vi "Get Meter Selected.vi"(0 "VISA resource name":refnum<visa-resource-name>, 11 "error in (no error)":errorcluster) -> (4 "VISA resource name out":refnum<visa-resource-name>, 6 "Meter Selected":u16(ring) items=["Frequency", "Peak Current", "Power", "Current", "Power Factor"], 15 "error out":errorcluster)   [LabVIEW 2020, in "eec 6700.lvlib"]
doc: "Gets the current meter selected in the power source instrument."
uses:
  <instrlib>/eec 6700/eec 6700.lvlib
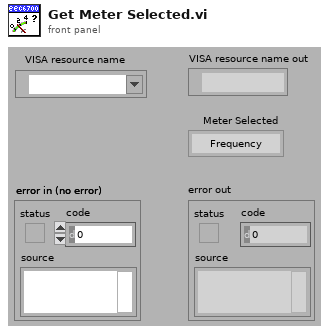
[diagram p1: front panel]
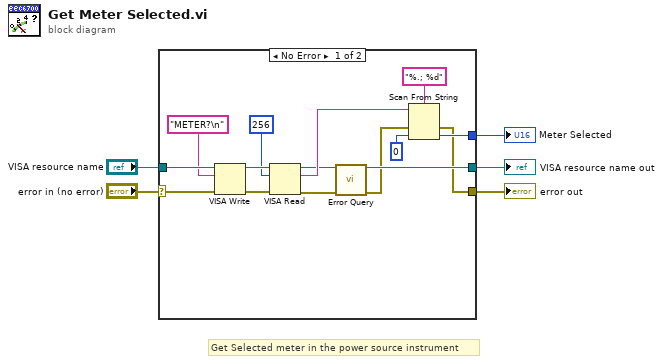
[diagram p0: block diagram]
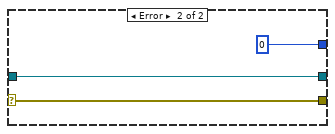
[diagram p2: hidden frame]
diagram:
  # "Get Selected meter in the power source instrument"
  n1 = case shown="No Error" "error in (no error)" {
    selector: "error in (no error)" -> [w11 w23]
    tunnel: "VISA resource name" -> [w20 w22]
    tunnel: [w10 w22] -> w4
    tunnel: [w8 w23] -> w3
    tunnel: [w15 u16 0 ("default value 1")] -> w2
    frame No Error {
      n2 = VISA Write(VISA resource name=w20, write buffer="METER?\n" ("command"), error in (no error)=w11) -> (VISA resource name out=w19:refnum<visa-resource-name>, error out=w18:errorcluster)  [unwired: 1 out]
      n3 = VISA Read(VISA resource name=w19, byte count=u32 256, error in (no error)=w18) -> (VISA resource name out=w9:refnum<visa-resource-name>, read buffer=w12:string, error out=w6:errorcluster)  [unwired: 1 out]
      n4 = call <instrlib>:"Error Query.vi"("VISA resource name"=w9, "error in (no error)"=w6) -> ("VISA resource name out"=w10:refnum<visa-resource-name>, "error out"=w7:errorcluster)  [unwired: 10 in, 2 out]
      n5 = Scan From String(format string="%.; %d", input string=w12, error in=w7, default 1=u16 0 ("default value 1")) -> (error out=w8:errorcluster, output 1=w15:u16)  [unwired: 1 in, 2 out]
    }
    frame Error {
    }
  }
  "VISA resource name out" <- w4
  "error out" <- w3
  "Meter Selected" <- w2
